vi "test Calculate Distance To Tag Within DistanceLimit.vi"(8 "error in (no error)":errorcluster, 11 "TestCase in":refnum<class "AnchorTests.lvclass">) -> (0 "error out":errorcluster, 3 "TestCase out":refnum<class "AnchorTests.lvclass">)   [LabVIEW 2014, in "AnchorTests.lvclass"]
uses:
  AnchorTests.lvclass
  <vilib>/addons/_JKI Toolkits/VI Tester/TestCase.llb/TestCase.lvclass
  SPLAT/Anchor/Anchor.lvclass
  SPLAT/Tag.lvclass
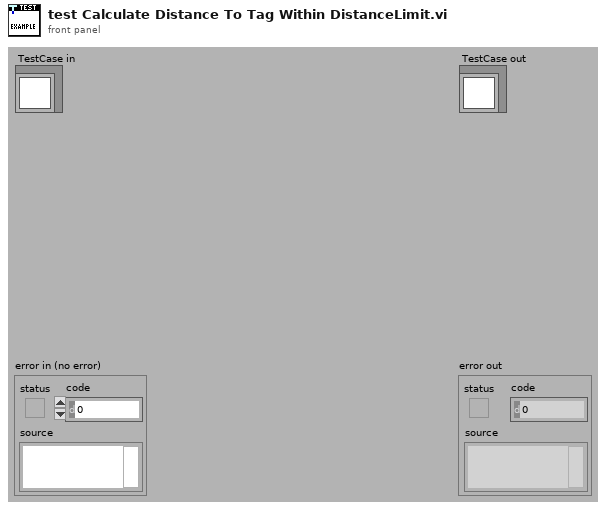
[diagram p1: front panel]
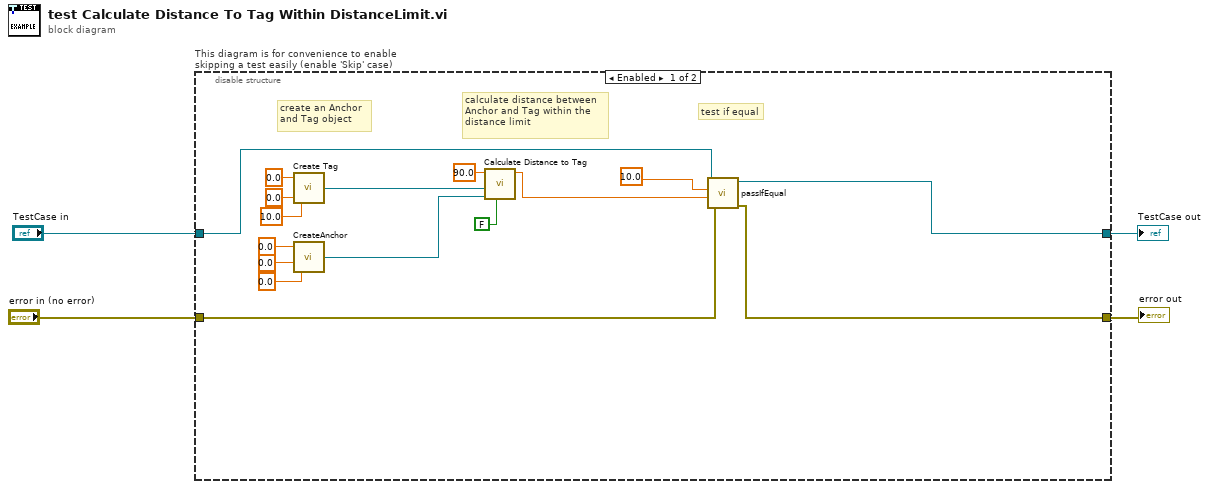
[diagram p0: block diagram]
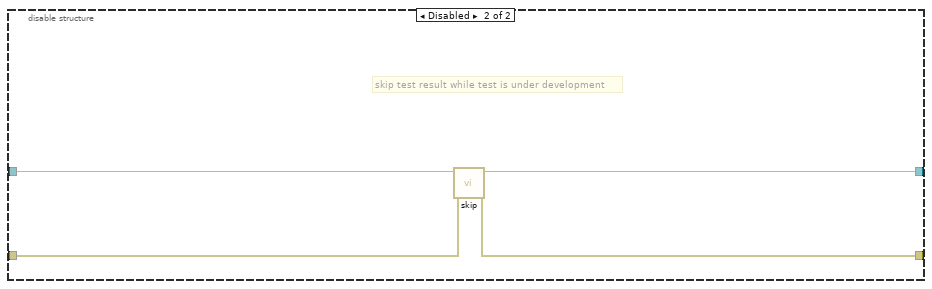
[diagram p2: hidden frame]
diagram:
  n1 = disable-structure "This diagram is for convenience to enable skipping a test easily (enable 'Skip' case)" shown="Enabled" {
    disable-tunnel: "TestCase in" -> [w10 w24]
    disable-tunnel: [w9 w22] -> w1
    disable-tunnel: [w8 w23] -> w3
    disable-tunnel: "error in (no error)" -> [w7 w21]
    frame Enabled {
      # "test if equal"
      # "create an Anchor\nand Tag object"
      # "calculate distance between\nAnchor and Tag within the\ndistance limit"
      n2 = call "Create Tag.vi"("TagY"=10.0, "TagX"=0.0, "TagID"=0.0) -> ("Tag Out"=w13:refnum<class "Tag.lvclass">)
      n3 = call "CreateAnchor.vi"("Anchor Y"=0.0, "Anchor X"=0.0, "Anchor ID"=0.0) -> ("Anchor Out"=w12:refnum<class "Anchor.lvclass">)
      n4 = call "Calculate Distance to Tag.vi"("Enable error margin"=FALSE, "Anchor.lvclass In"=w12, "Tag.lvclass"=w13, "DistanceLimit"=90.0) -> ("Distance"=w11:dbl)  [unwired: 6 in, 1 out]
      n5 = call-dynamic "passIfEqual.vi"("error in (no error)"=w7, "y"=w11, "x"=10.0, "TestCase in"=w10) -> ("error out"=w8:errorcluster, "TestCase out"=w9:refnum<class "AnchorTests.lvclass">)  [unwired: 6 in]
    }
    frame Disabled {
      # "skip test result while test is under development"
      n6 = call <vilib>:"skip.vi"("error in (no error)"=w21, "TestCase in"=w24) -> ("error out"=w23:errorcluster, "TestCase out"=w22:refnum<class "AnchorTests.lvclass">)  [unwired: 8 in]
    }
  }
  "error out" <- w3
  "TestCase out" <- w1
